vi "RandomValue.vi"(1 "factor":dbl=256.0) -> (0 "random value":dbl)   [LabVIEW 2009]
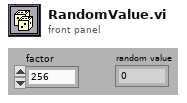
[diagram p1: front panel]
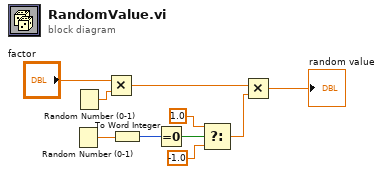
[diagram p0: block diagram]
diagram:
  n1 = Random Number (0-1)() -> (number: 0 to 1=w8:dbl)
  n2 = Random Number (0-1)() -> (number: 0 to 1=w10:dbl)
  n3 = Multiply(x="factor", y=w10) -> (x*y=w3:dbl)
  n4 = To Word Integer(number=w8) -> (16bit integer=w7:i16)
  n5 = Equal To 0?(x=w7) -> (x = 0?=w6:bool)
  n6 = Select(t=1.0 ("cas vrai"), s=w6, f=-1.0 ("cas faux")) -> (s? t:f=w2:dbl)
  n7 = Multiply(x=w3, y=w2) -> (x*y=→"random value":dbl)
